vi "Pitch Roll Control.vi"(0 "Left Motor In":dbl, 1 "Positive (Reverse) \nPitch Limit":dbl, 2 "Roll Limit":dbl, 3 "Right Motor In":dbl, 4 "Negative (Forward) \nPitch Limit":dbl) -> (5 "Roll":dbl, 6 "Left Motor Out":dbl, 7 "Case":i32, 8 "Pitch":dbl, 9 "Right Motor Out":dbl)   [LabVIEW 2013]
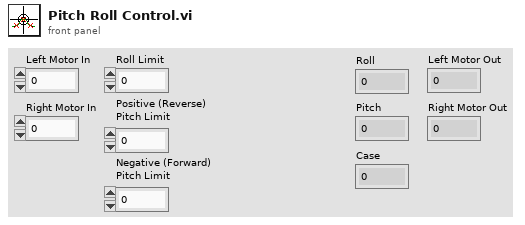
[diagram p1: front panel]
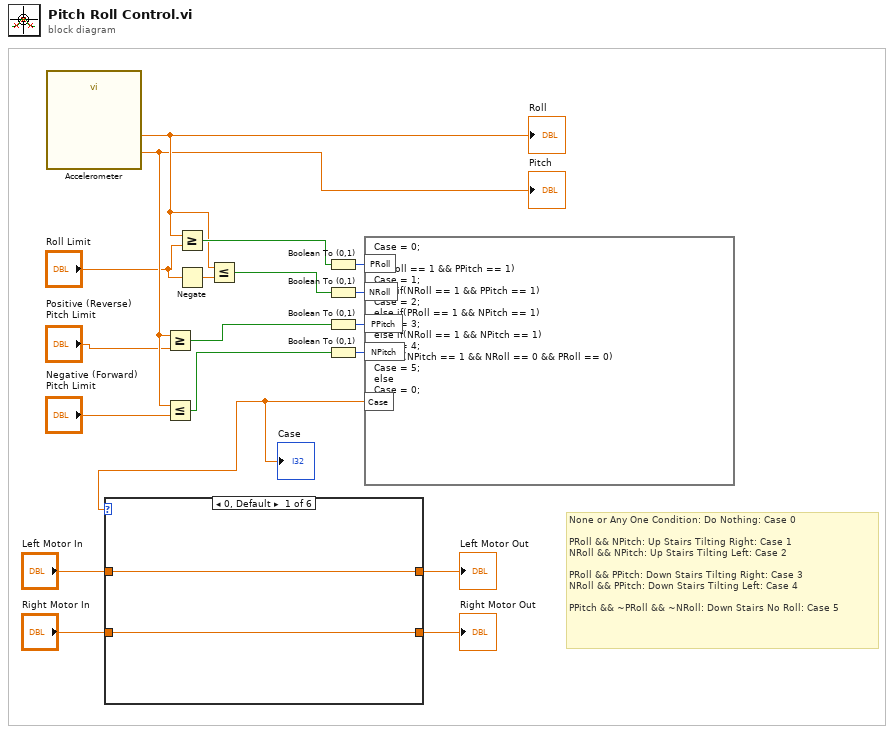
[diagram p0: block diagram]
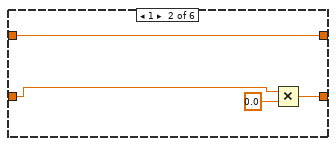
[diagram p2: hidden frame]
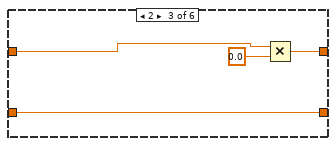
[diagram p3: hidden frame]
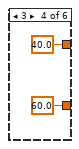
[diagram p4: hidden frame]
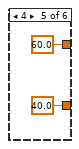
[diagram p5: hidden frame]
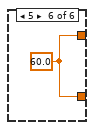
[diagram p6: hidden frame]
diagram:
  # "None or Any One Condition: Do Nothing: Case 0\n\nPRoll && NPitch: Up Stairs Tilting Right: Case 1\nNRoll && NPitch: Up Stairs Tilting Left: Case 2\n\nPRoll && PPitch: Down Stairs Tilting Right: Case 3\nNRoll && PPitch: Down Stairs Tilting Left: Case 4\n\nPPitch && ~PRoll && ~NRoll: Down Stairs No Roll: Case 5"
  n1 = call "Accelerometer"() -> ("Roll"=w9:dbl, "Pitch"=w6:dbl)  [unwired: 25 in, 1 out]
  "Roll" <- w9
  "Pitch" <- w6
  n2 = Greater Or Equal?(x=w6, y="Positive (Reverse) \nPitch Limit") -> (x >= y?=w7:bool)
  n3 = Less Or Equal?(x=w6, y="Negative (Forward) \nPitch Limit") -> (x <= y?=w5:bool)
  n4 = Greater Or Equal?(x=w9, y="Roll Limit") -> (x >= y?=w10:bool)
  n5 = Negate(x="Roll Limit") -> (-x=w3:dbl)
  n6 = Less Or Equal?(x=w9, y=w3) -> (x <= y?=w8:bool)
  n7 = Boolean To (0,1)(Boolean=w10) -> (0, 1=w12:i16)
  n8 = Boolean To (0,1)(Boolean=w8) -> (0, 1=w11:i16)
  n9 = Boolean To (0,1)(Boolean=w7) -> (0, 1=w14:i16)
  n10 = Boolean To (0,1)(Boolean=w5) -> (0, 1=w13:i16)
  n11 = formula code="Case = 0;\n\nif(PRoll == 1 && PPitch == 1) \nCase = 1;\nelse if(NRoll == 1 && PPitch == 1) \nCase = 2;\nelse if(PRoll == 1 && NPitch == 1) \nCase = 3;\nelse if(NRoll == 1 && NPitch == 1) \nCase = 4;\nelse if(NPitch == 1 && NRoll == 0 && PRoll == 0) \nCase = 5;\nelse \nCase = 0;"("PRoll"=w12, "NRoll"=w11, "PPitch"=w14, "NPitch"=w13) -> ("Case"=w15:dbl)
  "Case" <- w15
  n12 = case shown="0, Default" w15 {
    tunnel: "Left Motor In" -> [w21 w22 w28 _ _ _]
    tunnel: "Right Motor In" -> [w20 w23 w26 _ _ _]
    tunnel: [w21 w22 w27 40.0 ("Left Motor In") 60.0 ("Left Motor In") w34] -> w17
    tunnel: [w20 w25 w26 60.0 ("Right Motor In") 40.0 ("Right Motor In") w34] -> w16
    frame 0, Default {
    }
    frame 1 {
      n13 = Multiply(x=w23, y=0.0) -> (x*y=w25:dbl)
    }
    frame 2 {
      n14 = Multiply(x=w28, y=0.0) -> (x*y=w27:dbl)
    }
    frame 3 {
    }
    frame 4 {
    }
    frame 5 {
      w34 = 60.0
    }
  }
  "Left Motor Out" <- w17
  "Right Motor Out" <- w16
